vi "Conversor C a F-1-4.vi"(1 "Temperatura a convertir":dbl) -> (0 "Temp Convertida a C":dbl)   [LabVIEW 2013]
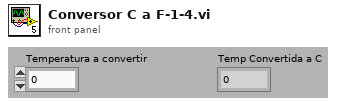
[diagram p1: front panel]
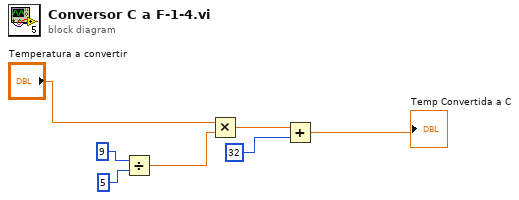
[diagram p0: block diagram]
diagram:
  n1 = Divide(x=9, y=5) -> (x/y=w2:dbl)
  n2 = Multiply(x="Temperatura a convertir", y=w2) -> (x*y=w7:dbl)
  n3 = Add(x=w7, y=32) -> (x+y=→"Temp Convertida a C":dbl)
